vi "Write CAN.vi"(4 "timeout":i32=1000, 6 "CAN Frame":T2={"Timestamp"=0, "Identifier"=0, "Type"=0, "InfoA"=0, "InfoB"=0, "DataLength"=0, "Data"=[0, 0, 0, 0, 0, 0, 0, 0]} {"Data" format="%.0x"; "DataLength" format="%.0x"; "InfoB" format="%.0x"; "InfoA" format="%.0x"; "Type" format="%.0x"; "Identifier" format="%.0x"; "Timestamp" format="%.0x"}, 8 "error in":errorcluster, 11 "CAN Session In":T1) -> (0 "error out":errorcluster, 3 "CAN Session Out":T1)   [LabVIEW 2016]
doc: "The VI writes a CAN packet (frame) to the write queue which results in that packet being written to the CAN bus."
uses:
  Typedefs/FPGA CAN Frame Cluster.ctl
  Typedefs/CAN Refnum.ctl
  Typedefs/CAN Session Pointer.ctl
  Typedefs/CAN Communication References.ctl
  Typedefs/kill process notifier array.ctl
  Typedefs/Write Queue.ctl
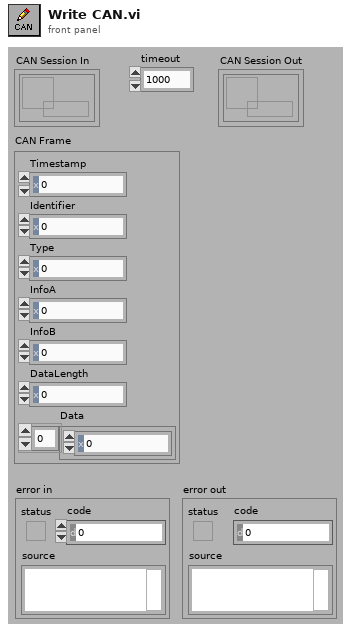
[diagram p1: front panel]
types:
  T1 = typedef "CAN Refnum.ctl" = refnum<k1>
  T2 = typedef "FPGA CAN Frame Cluster.ctl" = cluster{"Timestamp":u64, "Identifier":u32, "Type":u8, "InfoA":u8, "InfoB":u8, "DataLength":u8, "Data":u8[]}
  T3 = typedef "Write Queue.ctl" = refnum<queue>
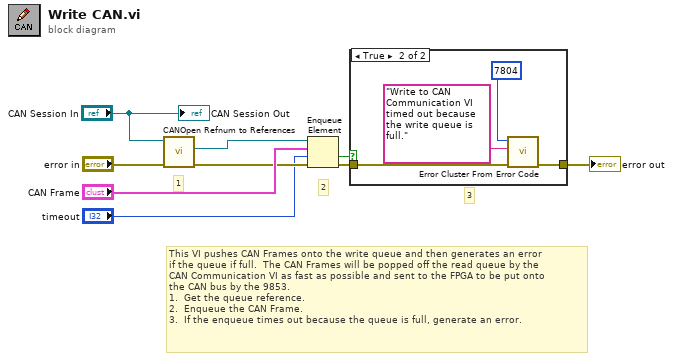
[diagram p0: block diagram]
diagram:
  # "3"
  # "2"
  # "1"
  # "This VI pushes CAN Frames onto the write queue and then generates an error\nif the queue if full.  The CAN Frames will be popped off the read queue by the\nCAN Communication VI as fast as possible and sent to the FPGA to be put onto\nthe CAN bus by the 9853.\n1.  Get the queue reference.\n2.  Enqueue the CAN Frame.\n3.  If the enqueue times out because the queue is full, generate an error."
  n1 = call "CANOpen Refnum to References.vi"("error in (no error)"="error in", "CAN Session In"="CAN Session In") -> ("error out"=w7:errorcluster, "Write Queue"=w6:T3)  [unwired: 8 out]
  n2 = Enqueue Element(queue=w6, element="CAN Frame", timeout in ms (-1)="timeout", error in (no error)=w7) -> (timed out?=w3:bool, error out=w2:errorcluster)  [unwired: 1 out]
  n3 = case shown="True" w3 {
    tunnel: w2 -> [w10 w14]
    tunnel: [w10 w13] -> w1
    frame False {
    }
    frame True {
      n4 = call <vilib>:"Error Cluster From Error Code.vi"("error in (no error)"=w14, "error message (\"\")"="Write to CAN Communication VI timed out because the write queue is full." ("error message (\"\")"), "error code (0)"=7804) -> ("error out"=w13:errorcluster)  [unwired: 1 in, 5 out]
    }
  }
  "error out" <- w1
  "CAN Session Out" <- "CAN Session In"
